vi "Global P.vi"() -> ()   [LabVIEW 2013]
panel:
  out "P":cluster{" P sens 1":dbl, "P sens 2":dbl}
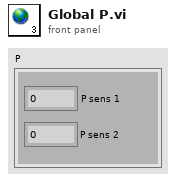
[diagram p1: front panel]
diagram:
